vi "Return to Thread Pool.vi"(8 "error in (no error)":errorcluster, 10 "Transfer Group in":refnum<class "Transfer Group.lvclass">, 11 "Plugin Thread in":refnum<class "Plugin Thread.lvclass">) -> (0 "error out":errorcluster, 3 "Plugin Thread out":refnum<class "Plugin Thread.lvclass">)   [LabVIEW 2017, in "DSF Core.lvlib" / "Plugin Thread.lvclass"]
uses:
  Thread/Plugin/Plugin Thread.lvclass
  Transfer Group/Transfer Group.lvclass
  Thread/Plugin/Plugin Thread.lvclass/Plugin Thread.ctl
  Pool/Plugin Interface/Plugin Interface Pool.lvclass
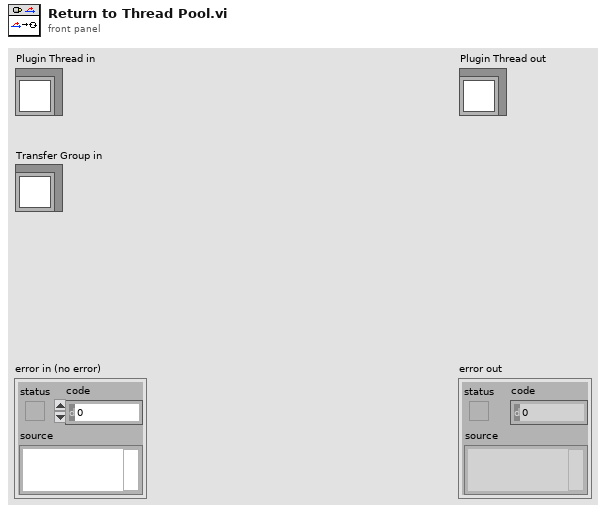
[diagram p1: front panel]
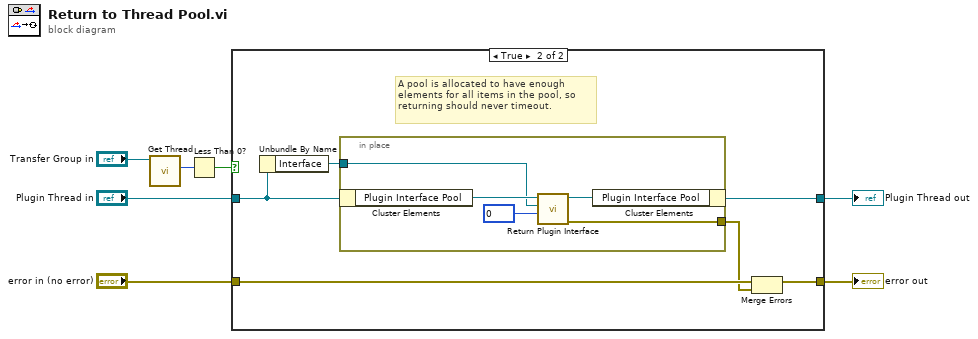
[diagram p0: block diagram]
diagram:
  n1 = call "Get Thread.vi"("Transfer Group in"="Transfer Group in") -> ("thread"=w3:i32)  [unwired: 9 in, 1 out]
  n2 = Less Than 0?(x=w3) -> (x < 0?=w2:bool)
  n3 = case shown="True" w2 {
    tunnel: [w8 w10] -> w7
    tunnel: "Plugin Thread in" -> [w9 w15]
    tunnel: [w9 w13] -> w5
    tunnel: "error in (no error)" -> [w8 w12]
    frame False {
      # "Thread is 0 or greater, meaning this thread was manually dispatched to, so don't return to thread pool."
    }
    frame True {
      # "A pool is allocated to have enough elements for all items in the pool, so returning should never timeout."
      n4 = Unbundle By Name(w15) -> ("Interface"=w14:refnum<class "Plugin Interface.lvclass">)
      n5 = in-place {
        in-place-border: [w20] -> w11
        in-place-border: w14 -> [w17]
        n6 = in-place-cluster #1(w15) -> ("Plugin Interface Pool"=w19:refnum<class "Plugin Interface Pool.lvclass">)
        n7 = call "Return Plugin Interface.vi"("timeout in ms (0)"=0, "Plugin Interface"=w17, "Plugin Interface Pool in"=w19) -> ("error out"=w20:errorcluster, "Plugin Interface Pool out"=w18:refnum<class "Plugin Interface Pool.lvclass">)  [unwired: 6 in, 1 out]
        n8 = in-place-cluster #1("Plugin Interface Pool"=w18) -> (w13:refnum<class "Plugin Thread.lvclass">)
      }
      n9 = Merge Errors(w12, w11) -> (w10:errorcluster)
    }
  }
  "error out" <- w7
  "Plugin Thread out" <- w5
